vi "AddS-Go-Get.vi"(5 "Channels":i32[](array[numeric]), 7 "IOTypes":string[](array[string]), 8 "error in":errorcluster, 9 "x1":i32[](array[numeric]), 10 "Values Write":dbl[](array[numeric]) format="%.2f", 11 "Handle In":i32) -> (0 "error out":errorcluster, 2 "Values Read":dbl[](array[numeric]) format="%.6f", 3 "Handle Out":i32)   [LabVIEW 2021]
doc: "This utility VI is an alternative to calling eAddGoGet from the UD libary.\nThe utility VI has better/easier error handling and is normally preferred in LabVIEW,\nbut eAddGoGet is a single call to the UD driver so often preferred if you will have\nparallel driver calls within the same thread."
panel:
  # "This utility VI is an alternative to calling eAddGoGet from the UD libary.\nThe utility VI has better/easier error handling and is normally preferred in LabVIEW,\nbut eAddGoGet is a single call to the UD driver so often preferred if you will have\nparallel driver calls within the same thread."
  # "Pass an array of IOTypes, and also pass arrays of\nchannels/values/x1 with elements for each\nIOType.  The size of the \"IOTypes\" array\ndetermines how many AddRequests are done."
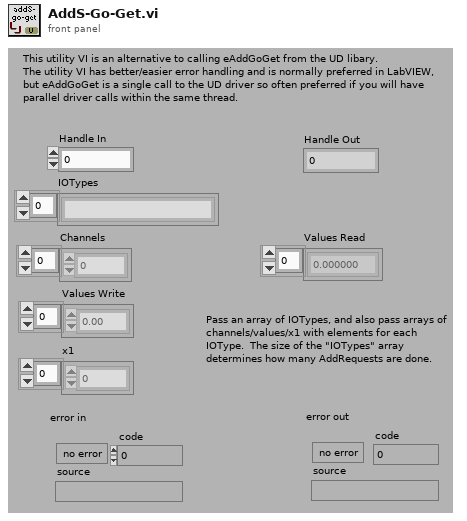
[diagram p1: front panel]
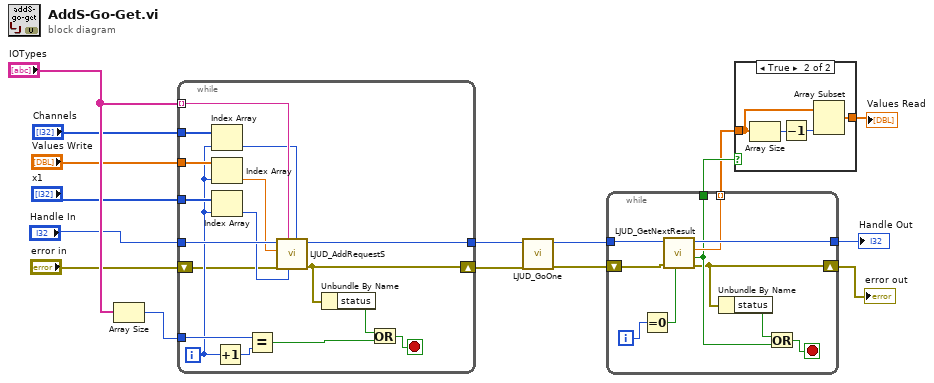
[diagram p0: block diagram]
diagram:
  n1 = Array Size(array="IOTypes") -> (size(s)=w16:i32)
  n2 = while {
    shift-left: "error in" -> [w18]
    shift-right: [w17] -> w3
    tunnel: "x1" -> [w25]
    tunnel: [w27] -> w11
    tunnel: "Handle In" -> [w28]
    tunnel: "Channels" -> [w23]
    tunnel: "Values Write" -> [w24]
    tunnel: "IOTypes" -> [w26] mode=indexing
    tunnel: w16 -> [w30]
    i -> [w22]
    stop <- w33 stop-if-true
    n3 = Index Array(array=w23, index=w22) -> (element=w21:i32)
    n4 = Index Array(array=w24, index=w22) -> (element=w20:dbl)
    n5 = Index Array(array=w25, index=w22) -> (element=w19:i32)
    n6 = Increment(x=w22) -> (x+1=w31:i32)
    n7 = Equal?(x=w30, y=w31) -> (x = y?=w29:bool)
    n8 = call "LJUD_AddRequestS.vi"("Channel"=w21, "x1"=w19, "IOType"=w26, "error in"=w18, "Value"=w20, "Handle In"=w28) -> ("error out"=w17:errorcluster, "Handle Out"=w27:i32)  [unwired: 4 in]
    n9 = Unbundle By Name(w17) -> ("status"=w32:bool)
    n10 = Or(x=w32, y=w29) -> (x .or. y?=w33:bool)
  }
  n11 = call "LJUD_GoOne.vi"("error in"=w3, "Handle In"=w11) -> ("error out"=w2:errorcluster, "Handle Out"=w10:i32)  [unwired: 8 in]
  n12 = while {
    shift-left: w2 -> [w35]
    shift-right: [w34] -> w1
    tunnel: [w36] -> w8
    tunnel: [w37] -> w7 mode=indexing
    tunnel: [w39] -> w9
    tunnel: w10 -> [w41]
    i -> [w38]
    stop <- w43 stop-if-true
    n13 = Equal To 0?(x=w38) -> (x = 0?=w42:bool)
    n14 = call "LJUD_GetNextResult.vi"("GetFirst"=w42, "error in"=w35, "Handle In"=w41) -> ("error out"=w34:errorcluster, "LJE_NO_MORE_DATA_AVAILABLE"=w36:bool, "Value"=w37:dbl, "Handle Out"=w39:i32)  [unwired: 3 in, 2 out]
    n15 = Unbundle By Name(w34) -> ("status"=w40:bool)
    n16 = Or(x=w40, y=w36) -> (x .or. y?=w43:bool)
  }
  "Handle Out" <- w9
  "error out" <- w1
  n17 = case shown="True" w8 {
    tunnel: w7 -> [w44 w46]
    tunnel: [w44 w45] -> w6
    frame False {
    }
    frame True {
      n18 = Array Size(array=w46) -> (size(s)=w48:i32)
      n19 = Decrement(x=w48) -> (x-1=w47:i32)
      n20 = Array Subset(array=w46, length=w47) -> (w45:dbl[])  [unwired: 1 in]
    }
  }
  "Values Read" <- w6
